vi "Read Nested Models.vi"(11 "Launch Nested Models Msg":refnum<class "Launch Nested Models Msg.lvclass">) -> (2 "Nested Models":refnum<class "IModel.lvclass">[](array[class]))   [LabVIEW 2017, in "IModel.lvlib" / "Launch Nested Models Msg.lvclass"]
uses:
  Launch Nested Models Msg.lvclass
  IModel/IModel.lvclass
  Launch Nested Models Msg.lvclass/Launch Nested Models Msg.ctl
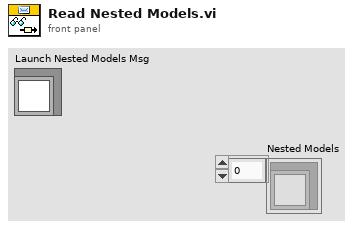
[diagram p1: front panel]
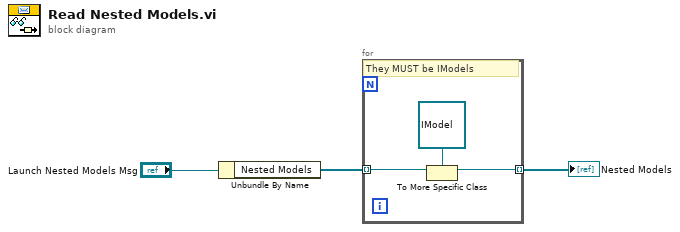
[diagram p0: block diagram]
diagram:
  n1 = Unbundle By Name("Launch Nested Models Msg") -> ("Nested Models"=w2:refnum<class "Actor.lvclass">[])
  n2 = for {
    tunnel: w2 -> [w6] mode=indexing
    tunnel: [w5] -> w1 mode=indexing
    # "They MUST be IModels"
    n3 = To More Specific Class(target class=refnum<class "IModel.lvclass"> refnum ("IModel.lvlib:IModel.lvclass"), reference=w6) -> (specific class reference=w5:refnum<class "IModel.lvclass">)  [unwired: 1 in, 1 out]
  }
  "Nested Models" <- w1
